vi "Pre Launch Init.vi"(11 "MQTT-Server in":refnum<class "MQTT-Server.lvclass">) -> (0 "error out":errorcluster, 3 "MQTT-Server out":refnum<class "MQTT-Server.lvclass">)   [LabVIEW 2023, in "MQTT-Server.lvlib" / "MQTT-Server.lvclass"]
doc: "(<B>Filename</B>: Actor Framework.lvlib:Actor.lvclass:Pre Launch Init.vi)\n\nDefines behavior that occurs after the Launch Nested Actor method is invoked but before the actor's Actor Core method begins running.\n\nBy default, this method does nothing. A descendant class may override it to define behavior."
uses:
  MQTT-Server.lvclass
  MQTT-Server.lvclass/MQTT-Server.ctl
  <vilib>/ActorFramework/Actor/Actor.lvclass
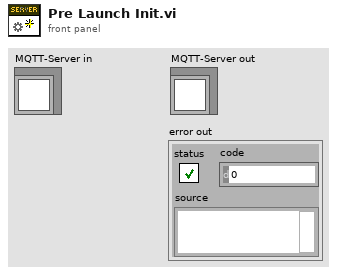
[diagram p1: front panel]
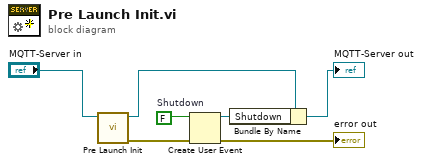
[diagram p0: block diagram]
diagram:
  w6 = FALSE  # Shutdown
  n1 = call-parent "Pre Launch Init.vi"("Actor in"="MQTT-Server in") -> ("error out"=w5:errorcluster, "Actor out"=w3:refnum<class "MQTT-Server.lvclass">)  [unwired: 9 in]
  n2 = Create User Event(user event datatype=w6, error in=w5) -> (user event=w2:refnum<user-event>, error out=→"error out":errorcluster)
  n3 = Bundle By Name(cluster=w3, "Shutdown"=w2) -> (→"MQTT-Server out":refnum<class "MQTT-Server.lvclass">)
